vi "PWM lenkberechnung.vi"(0 "wert vorne":dbl, 1 "gewicht vorne":dbl, 2 "wert schräg":dbl, 3 "gewicht schräg":dbl, 4 "wert seiten":dbl, 5 "gewicht seiten":dbl) -> (16 "ausgabe zu pide":dbl)   [LabVIEW 2016]
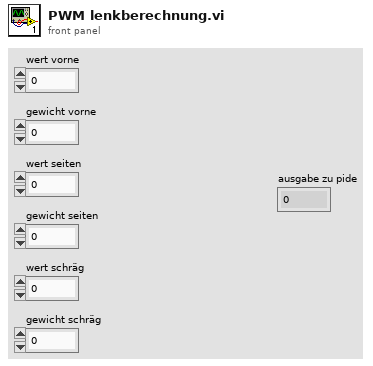
[diagram p1: front panel]
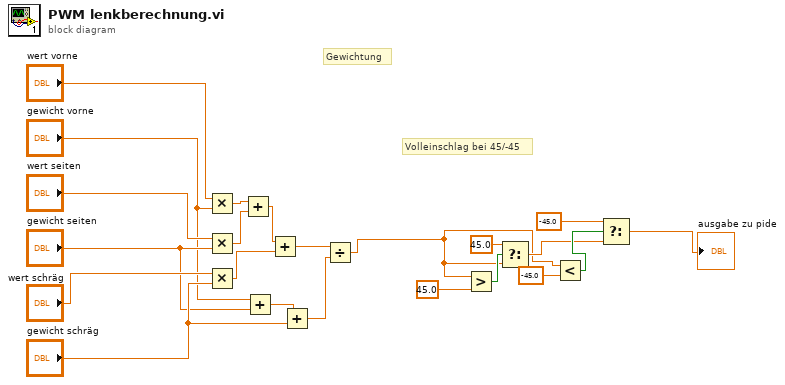
[diagram p0: block diagram]
diagram:
  # "Volleinschlag bei 45/-45"
  # "Gewichtung"
  n1 = Multiply(x="wert vorne", y="gewicht vorne") -> (x*y=w22:dbl)
  n2 = Multiply(x="wert seiten", y="gewicht seiten") -> (x*y=w15:dbl)
  n3 = Multiply(x="wert schräg", y="gewicht schräg") -> (x*y=w17:dbl)
  n4 = Add(x=w22, y=w15) -> (x+y=w21:dbl)
  n5 = Add(x="gewicht vorne", y="gewicht seiten") -> (x+y=w19:dbl)
  n6 = Add(x=w21, y=w17) -> (x+y=w20:dbl)
  n7 = Add(x=w19, y="gewicht schräg") -> (x+y=w18:dbl)
  n8 = Divide(x=w20, y=w18) -> (x/y=w2:dbl)
  n9 = Greater?(x=w2, y=45.0) -> (0:w9:bool)
  n10 = Select(t=45.0, s=w9, f=w2) -> (s? t:f=w3:dbl)
  n11 = Less?(x=w2, y=-45.0) -> (x < y?=w4:bool)
  n12 = Select(t=-45.0, s=w4, f=w3) -> (s? t:f=→"ausgabe zu pide":dbl)
